vi "DFD Integer Delay (PtByPt NChan).vi"(7 "init? (F)":bool, 8 "error in (no error)":errorcluster, 10 "delay":i32, 11 "signal in":dbl[](array[numeric])) -> (0 "error out":errorcluster, 3 "signal out":dbl[](array[numeric]))   [LabVIEW 2017, in "NI_DigFilterLicensed.lvlib"]
doc: "Delays a signal continuously by a specified integer number of sample intervals. Wire data to the <B>signal in</B> input to determine the polymorphic instance to use or manually select the instance."
uses:
  <vilib>/addons/Digital Filter Design/NI_DigFilterLicensed.lvlib
  <vilib>/addons/Digital Filter Design/Process.llb/DFD Integer Delay with State (PtByPt).vi
  <vilib>/addons/Digital Filter Design/NI_DigFilter_Process.lvlib
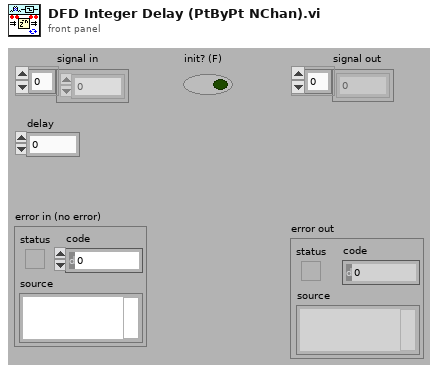
[diagram p1: front panel]
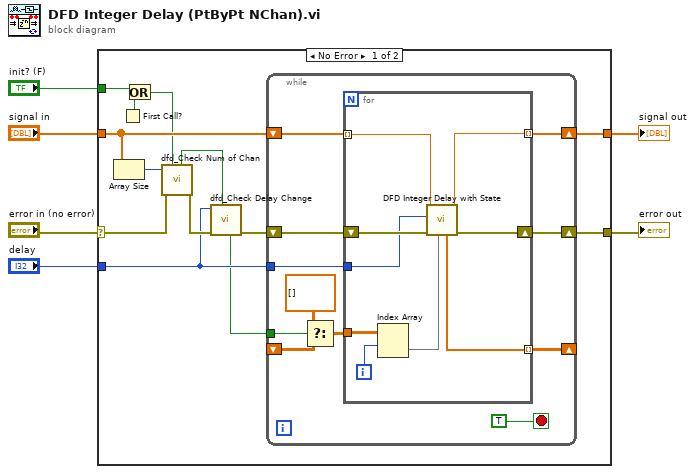
[diagram p0: block diagram]
diagram:
  n1 = case shown="No Error" "error in (no error)" {
    selector: "error in (no error)" -> [w12 w40]
    tunnel: [w19 w40] -> w6
    tunnel: "signal in" -> [w15 _]
    tunnel: [w18 _] -> w4
    tunnel: "delay" -> [w9 _]
    tunnel: "init? (F)" -> [w16 _]
    frame No Error {
      n2 = Array Size(array=w15) -> (size(s)=w14:i32)
      n3 = First Call?() -> (First Call?: T/F=w17:bool)
      n4 = Or(x=w16, y=w17) -> (x .or. y?=w13:bool)
      n5 = call <vilib>:"dfd_Check Num of Chan.vi"("init in"=w13, "error in (no error)"=w12, "#ch in"=w14) -> ("error out"=w11:errorcluster, "init out"=w8:bool)  [unwired: 7 out]
      n6 = call <vilib>:"dfd_Check Delay Change.vi"("init in"=w8, "error in (no error)"=w11, "delay in"=w9) -> ("error out"=w10:errorcluster, "init out"=w7:bool)  [unwired: 7 out]
      n7 = while {
        shift-right: [w29] -> _
        shift-left: _ -> [w27]
        tunnel: w7 -> [w22]
        tunnel: w9 -> [w23]
        shift-right: [w24] -> w18
        shift-left: w15 -> [w25]
        shift-right: [w21] -> w19
        shift-left: w10 -> [w28]
        stop <- TRUE stop-if-true
        n8 = Select(t=dbl[][] [], s=w22, f=w27) -> (s? t:f=w26:dbl[][])
        n9 = for {
          tunnel: [w39] -> w29 mode=indexing
          tunnel: w26 -> [w36]
          tunnel: w25 -> [w34] mode=indexing
          tunnel: [w33] -> w24 mode=indexing
          tunnel: w23 -> [w32]
          shift-right: [w37] -> w21
          shift-left: w28 -> [w38]
          i -> [w31]
          n10 = Index Array(array=w36, index (row)=w31) -> (element=w35:dbl[])  [unwired: 1 in]
          n11 = call-poly <vilib>:"DFD Integer Delay with State.vi"("state in"=w35, "error in (no error)"=w38, "delay"=w32, "signal in"=w34) -> ("error out"=w37:errorcluster, "signal out"=w33:dbl, "state out"=w39:dbl[])  [unwired: 5 out]
        }
      }
    }
    frame Error {
    }
  }
  "error out" <- w6
  "signal out" <- w4
